vi "15.3 Golden Template Inspection.vi"() -> ()   [LabVIEW 2016]
doc: "This example shows how to use the Golden Template Inspection VIs in NI Vision.\n\nThe example locates the object for inspection (a printed label) in the inspected image using Pattern Matching. Then the example compares a printed label with no defects (the golden template) with the inspected label. If the inspected label has any large defects, the label fails the inspection. The golden template file used in this example was created using the NI Vision Template Editor. The NI Vision Template Editor allows you to configure and then save information in a template file, such as the information this example used for Pattern Matching and Golden Template Inspection."
uses:
  <vilib>/vision/Inspection.llb/IMAQ Inspection Options.ctl
  <vilib>/vision/NI_Vision_Development_Module.lvlib
panel:
  in  "Defect Display Options":T1={"Show Bright Defects"=TRUE, "Bright Color"=6618880, "Show Dark Defects"=TRUE, "Dark Color"=16711680}
  out "Pass Status":bool
  out "UUT":T2(plugin-control)
  out "Golden Template":T2(plugin-control)
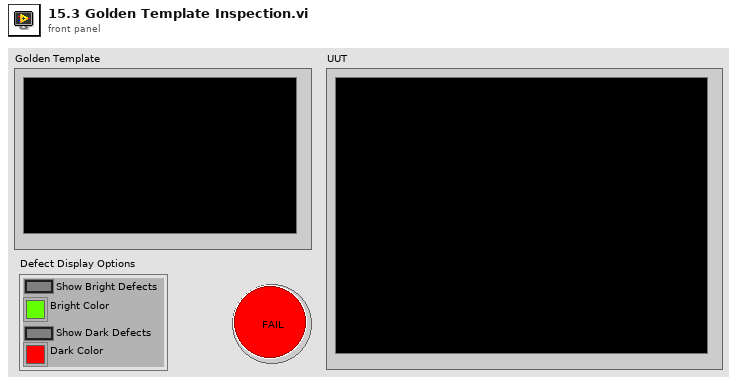
[diagram p1: front panel]
types:
  T1 = cluster{"Show Bright Defects":bool, "Bright Color":u32, "Show Dark Defects":bool, "Dark Color":u32}
  T2 = typedef "IMAQ Image.ctl" = refnum<image>
  T3 = cluster{"Number of Matches Requested":i32, "Minimum Match Score":sgl, "Angle Ranges":cluster{"Start Angle":sgl, "End Angle":sgl}[]}
  T4 = cluster{"Position":cluster{"x":sgl, "y":sgl}, "Angle":sgl, "Scale":sgl, "Score":sgl, "Bounding Box":cluster{"x":sgl, "y":sgl}[]}[]
  T5 = typedef "IMAQ Inspection Options.ctl" = cluster{"Registration Method":u32, "Normalization Method":u32, "Edge Thickness to Ignore":i32, "Bright Threshold":sgl, "Dark Threshold":sgl, "Grayscale/ Binary?":bool}
  T6 = cluster{"Position":cluster{"x":sgl, "y":sgl}, "Angle":sgl, "Scale":sgl, "Score":sgl, "Bounding Box":cluster{"x":sgl, "y":sgl}[]}
  T7 = cluster{"Position":cluster{"x":sgl, "y":sgl}, "Angle":sgl, "Scale":sgl}
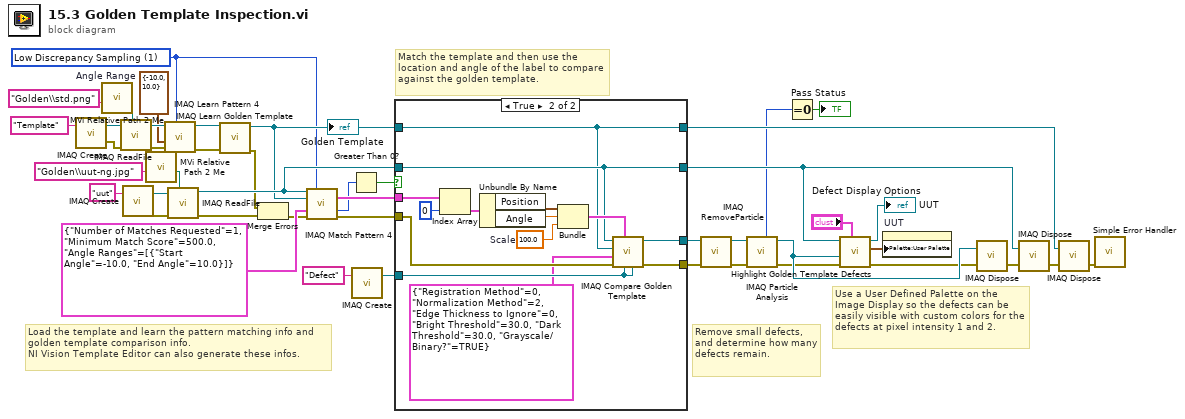
[diagram p0: block diagram]
diagram:
  w2 = cluster{"Start Angle":sgl, "End Angle":sgl} {"Start Angle"=-10.0, "End Angle"=10.0}  # Angle Range
  w1 = 1 items=["All", "Low Discrepancy Sampling", "Grayscale Value Pyramid", "Gradients Pyramid"] ("Algorithm")
  # "Use a User Defined Palette on the Image Display so the defects can be easily visible with custom colors for the defects at pixel intensity 1 and 2."
  # "Remove small defects, and determine how many defects remain."
  # "Load the template and learn the pattern matching info and golden template comparison info.\nNI Vision Template Editor can also generate these infos."
  # "Match the template and then use the location and angle of the label to compare against the golden template."
  n1 = call "IMAQ Create"("Image Name"="Template") -> ("Src"=w10:T2, "error out"=w11:errorcluster)  [unwired: 3 in, 1 out]
  n2 = call "MVi Relative Path 2 Me.vi"("Relative Path"="Golden\\std.png") -> ("Appended Dir"=w4:path)  [unwired: 5 in, 1 out]
  n3 = call "IMAQ ReadFile"("File Path"=w4, "error in (no error)"=w11, "Image"=w10) -> ("error out"=w9:errorcluster, "Image Out"=w8:T2)  [unwired: 4 in, 3 out]
  n4 = call "IMAQ Create"("Image Name"="uut") -> ("Src"=w25:T2, "error out"=w26:errorcluster)  [unwired: 3 in, 1 out]
  n5 = call "MVi Relative Path 2 Me.vi"("Relative Path"="Golden\\uut-ng.jpg") -> ("Appended Dir"=w24:path)  [unwired: 5 in, 1 out]
  n6 = call "IMAQ Learn Pattern 4"("Algorithm"=w1, "error in (no error)"=w9, "Angle Range"=w2, "Image"=w8) -> ("error out"=w13:errorcluster, "Template Image Out"=w12:T2)  [unwired: 5 in, 1 out]
  n7 = call "IMAQ ReadFile"("File Path"=w24, "error in (no error)"=w26, "Image"=w25) -> ("error out"=w6:errorcluster, "Image Out"=w21:T2)  [unwired: 4 in, 3 out]
  n8 = call "IMAQ Learn Golden Template"("error in (no error)"=w13, "Template"=w12) -> ("error out"=w7:errorcluster, "Template Out"=w3:T2)  [unwired: 8 in]
  "Golden Template" <- w3
  n9 = Merge Errors(w7, w6) -> (w5:errorcluster)
  n10 = call "IMAQ Match Pattern 4"("Image"=w21, "Algorithm"=w1, "Template Image"=w3, "Parameters"=T3 {"Number of Matches Requested"=1, "Minimum Match Score"=500.0, "Angle Ranges"=[{"Start Angle"=-10.0, "End Angle"=10.0}]}, "error in (no error)"=w5) -> ("Matches (pixel)"=w19:T4, "Number of Matches"=w18:i32, "error out"=w20:errorcluster)  [unwired: 6 in, 2 out]
  n11 = Greater Than 0?(x=w18) -> (x > 0?=w34:bool)
  n12 = call "IMAQ Create"("Image Name"="Defect") -> ("Src"=w45:T2)  [unwired: 3 in, 2 out]
  n13 = case shown="True" w34 {
    tunnel: w20 -> [w49 w51]
    tunnel: w21 -> [w48 w54]
    tunnel: w3 -> [w47 w53]
    tunnel: w19 -> [_ w62]
    tunnel: w45 -> [w46 w52]
    tunnel: [w49 w60] -> w32
    tunnel: [w46 w55] -> w17
    tunnel: [w48 w54] -> w40
    tunnel: [w47 w53] -> w38
    frame False {
    }
    frame True {
      w57 = sgl 100.0  # Scale
      n14 = Index Array(array=w62, index=0) -> (element=w61:T6)
      n15 = Unbundle By Name(w61) -> ("Position"=w59:cluster{"x":sgl, "y":sgl}, "Angle"=w58:sgl)
      n16 = Bundle("Position"=w59, "Angle"=w58, "Scale"=w57) -> (w56:T7)  [unwired: 1 in]
      n17 = call "IMAQ Compare Golden Template"("Dark Defect Image Dst"=w52, "Bright (or Both) Defect Image Dst"=w52, "Alignment"=w56, "error in (no error)"=w51, "Inspection Options"=T5 {"Registration Method"=0, "Normalization Method"=2, "Edge Thickness to Ignore"=0, "Bright Threshold"=30.0, "Dark Threshold"=30.0, "Grayscale/ Binary?"=TRUE}, "Template Image"=w53, "Image"=w54) -> ("error out"=w60:errorcluster, "Bright (or Both) Defect Image Dst Out"=w55:T2)  [unwired: 3 out]
    }
  }
  n18 = call "IMAQ RemoveParticle"("error in (no error)"=w32, "Image Src"=w17) -> ("error out"=w31:errorcluster, "Image Dst Out"=w16:T2)  [unwired: 5 in, 3 out]
  n19 = call "IMAQ Particle Analysis"("error in (no error)"=w31, "Image"=w16) -> ("error out"=w29:errorcluster, "Image Out (duplicate)"=w42:T2, "Number of Particles"=w33:i32)  [unwired: 3 in, 4 out]
  n20 = Equal To 0?(x=w33) -> (x = 0?=→"Pass Status":bool)
  n21 = call "Highlight Golden Template Defects.vi"("Defect Display Options"="Defect Display Options", "error in (no error)"=w29, "Defect Image"=w42, "Source Image"=w40) -> ("error out"=w23:errorcluster, "User Defined Color Palette"=w30:cluster{"Red":u8, "Green":u8, "Blue":u8}[], "Image Out"=→"UUT":T2)  [unwired: 5 in]
  n22 = property on="UUT" class="ImageControl"("Palette:User Palette"=w30) -> ()  [unwired: 2 in, 2 out]
  n23 = call "IMAQ Dispose"("Image"=w42, "error in (no error)"=w23) -> ("error out"=w41:errorcluster)  [unwired: 4 in]
  n24 = call "IMAQ Dispose"("Image"=w40, "error in (no error)"=w41) -> ("error out"=w39:errorcluster)  [unwired: 4 in]
  n25 = call "IMAQ Dispose"("Image"=w38, "error in (no error)"=w39) -> ("error out"=w37:errorcluster)  [unwired: 4 in]
  n26 = call <vilib>:"Simple Error Handler.vi"("error in (no error)"=w37) -> ()  [unwired: 4 in, 5 out]
